vi "get start node.vi"(8 "error in (no error)":errorcluster, 10 "start node path (root)":string, 11 "abstract-tree in":refnum<class "abstract-tree.lvclass">) -> (0 "error out":errorcluster, 2 "start node":refnum<k24>, 3 "abstract-tree out":refnum<class "abstract-tree.lvclass">)   [LabVIEW 2017, in "vs-tree-utility.lvlib" / "abstract-tree.lvclass"]
uses:
  abstract-tree.lvclass
  NationalInstruments.VeriStand.SystemStorage
  abstract-tree.lvclass/abstract-tree.ctl
  NationalInstruments.VeriStand.SystemDefinitionAPI
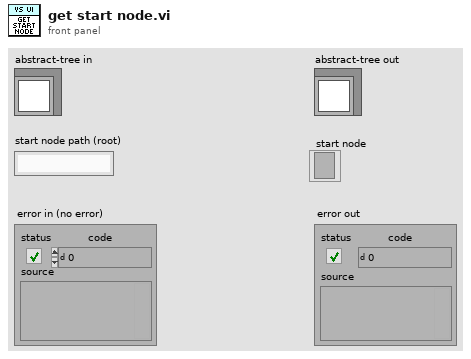
[diagram p1: front panel]
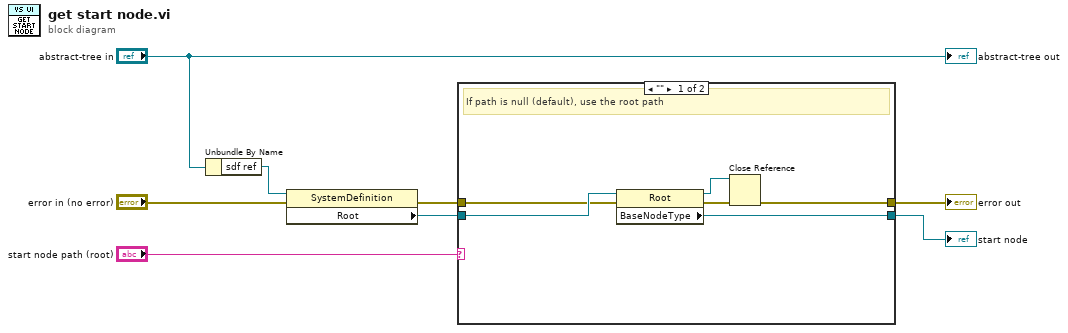
[diagram p0: block diagram]
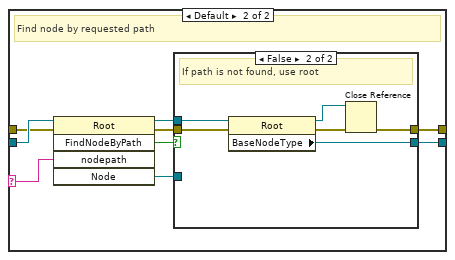
[diagram p2: hidden frame]
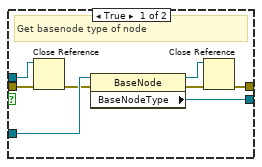
[diagram p3: hidden frame]
diagram:
  n1 = Unbundle By Name("abstract-tree in") -> ("sdf ref"=w2:refnum<k24>)
  n2 = property class="SystemDefinition"(reference=w2, error in="error in (no error)") -> (error out=w6:errorcluster, "Root"=w8:refnum<k24>)  [unwired: 1 out]
  n3 = case shown="\"\"" "start node path (root)" {
    selector: "start node path (root)" -> [_ w22]
    tunnel: w8 -> [w14 w23]
    tunnel: [w13 w20] -> w5
    tunnel: w6 -> [w12 w19]
    tunnel: [w10 w15] -> w3
    frame "" {
      # "If path is null (default), use the root path"
      n4 = property class="Root"(reference=w14, error in=w12) -> (reference out=w9:refnum<k24>, error out=w11:errorcluster, "BaseNodeType"=w13:refnum<k24>)
      n5 = Close Reference(reference=w9, error in (no error)=w11) -> (error out=w10:errorcluster)
    }
    frame Default {
      # "Find node by requested path"
      n6 = invoke class="Root" method="FindNodeByPath"(reference=w23, error in=w19, "nodepath"=w22) -> (reference out=w16:refnum<k24>, error out=w18:errorcluster, "FindNodeByPath"=w17:bool, "Node"=w21:refnum<k24>)  [unwired: 2 in, 1 out]
      n7 = case shown="False" w17 {
        tunnel: w21 -> [w31 _]
        tunnel: [w30 w37] -> w20
        tunnel: w18 -> [w29 w36]
        tunnel: w16 -> [w24 w35]
        tunnel: [w27 w33] -> w15
        frame True {
          # "Get basenode type of node"
          n8 = Close Reference(reference=w24, error in (no error)=w29) -> (error out=w25:errorcluster)
          n9 = property class="BaseNode"(reference=w31, error in=w25) -> (reference out=w26:refnum<k24>, error out=w28:errorcluster, "BaseNodeType"=w30:refnum<k24>)
          n10 = Close Reference(reference=w26, error in (no error)=w28) -> (error out=w27:errorcluster)
        }
        frame False {
          # "If path is not found, use root"
          n11 = property class="Root"(reference=w35, error in=w36) -> (reference out=w32:refnum<k24>, error out=w34:errorcluster, "BaseNodeType"=w37:refnum<k24>)
          n12 = Close Reference(reference=w32, error in (no error)=w34) -> (error out=w33:errorcluster)
        }
      }
    }
  }
  "error out" <- w3
  "start node" <- w5
  "abstract-tree out" <- "abstract-tree in"
